vi "ReadRealStatus气密机一.vi"(0 "从站地址":u8=255 format="%x", 5 "VISA":refnum<visa-resource-name>="COM3" caption="COM", 7 "baud rate":u32=57600 caption="波特率(9600)") -> (1 "Ready":bool, 2 "Pass":bool, 3 "StepCode":u16, 4 "ProgramNumber":u16, 6 "Pressure":dbl, 8 "PressureUnit":u16(ring) items=["cm3/s"=0, "cm3/min"=1000, "cm3/h"=2000, "mm3/h"=3000, "CalibartedPascal"=4000, "Pa"=6000, "Bar"=11000, "Kpa"=12000, "PSI"=13000, "Mbar"=14000, "Mpa"=15000, "Inch3/s"=46000, "Inch3/min"=47000, "Inch3/hour"=48000], 9 "AL":bool, 10 "Leak":dbl, 11 "PressureAL":bool, 12 "RD":bool, 13 "TD":bool, 14 "StatusResults":u16 format="%b", 15 "LeakUnit":u16(ring) items=["cm3/s"=0, "cm3/min"=1000, "cm3/h"=2000, "mm3/h"=3000, "CalibartedPascal"=4000, "Pa"=6000, "Bar"=11000, "Kpa"=12000, "PSI"=13000, "Mbar"=14000, "Mpa"=15000, "Inch3/s"=46000, "Inch3/min"=47000, "Inch3/hour"=48000])   [LabVIEW 2014]
panel:
  out "Read Status":bool
  out "ReturnResultValues":u16[](array[numeric]) format="%x"
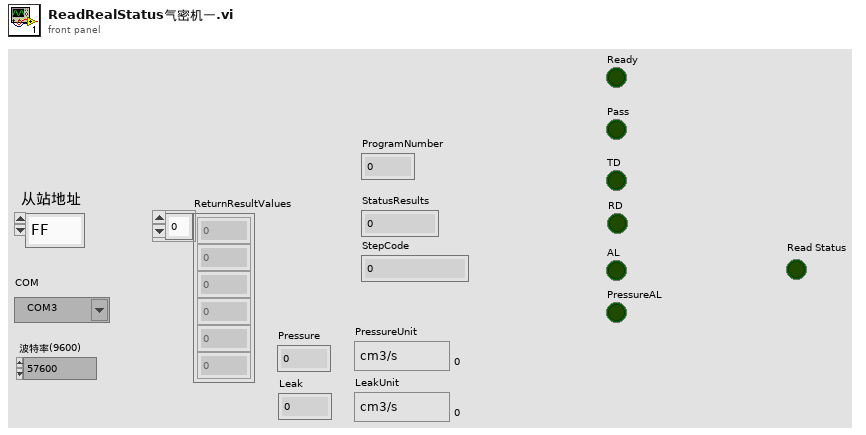
[diagram p1: front panel]
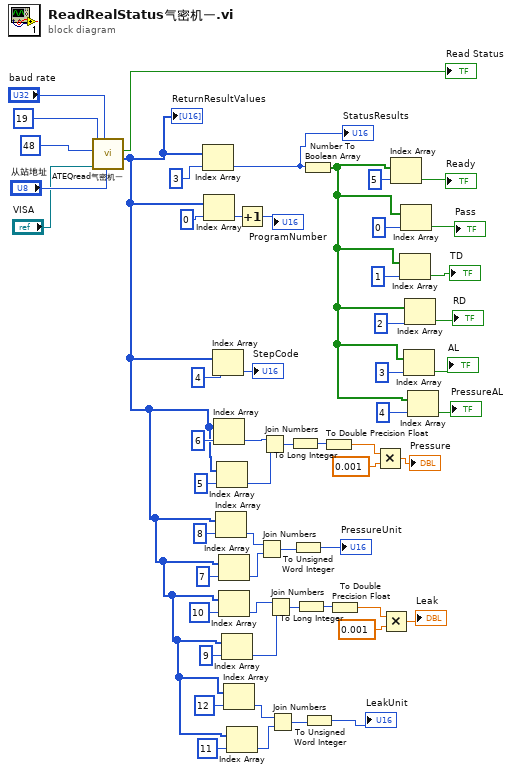
[diagram p0: block diagram]
diagram:
  n1 = call "ATEQread气密机一.vi"("baud rate (9600)"="baud rate", "VISA resource name"="VISA", "从站地址"="从站地址", "Read Address"=u16 48, "The number of Read"=u32 19) -> ("ReturnResultValues"=w12:u16[], "Read Status"=→"Read Status":bool)  [unwired: 4 in, 1 out]
  "ReturnResultValues" <- w12
  n2 = Index Array(array=w12, index=3 ("索引")) -> (element=w37:u16)
  "StatusResults" <- w37
  n3 = Index Array(array=w12, index=0 ("索引")) -> (element=w53:u16)
  n4 = Index Array(array=w12, index=4 ("索引")) -> (element=→"StepCode":u16)
  n5 = Index Array(array=w12, index=6 ("索引")) -> (element=w34:u16)
  n6 = Index Array(array=w12, index=8 ("索引")) -> (element=w26:u16)
  n7 = Index Array(array=w12, index=5 ("索引")) -> (element=w33:u16)
  n8 = Index Array(array=w12, index=7 ("索引")) -> (element=w25:u16)
  n9 = Index Array(array=w12, index=10 ("索引")) -> (element=w16:u16)
  n10 = Index Array(array=w12, index=9 ("索引")) -> (element=w15:u16)
  n11 = Index Array(array=w12, index=12 ("索引")) -> (element=w10:u16)
  n12 = Index Array(array=w12, index=11 ("索引")) -> (element=w9:u16)
  n13 = Increment(x=w53) -> (x+1=→"ProgramNumber":u16)
  n14 = Join Numbers(hi=w26, lo=w25) -> ((hi.lo)=w24:u32)
  n15 = Join Numbers(hi=w34, lo=w33) -> ((hi.lo)=w32:u32)
  n16 = Join Numbers(hi=w16, lo=w15) -> ((hi.lo)=w17:u32)
  n17 = Join Numbers(hi=w10, lo=w9) -> ((hi.lo)=w11:u32)
  n18 = To Long Integer(number=w32) -> (32bit integer=w31:i32)
  n19 = To Unsigned Word Integer(number=w24) -> (unsigned 16bit integer=→"PressureUnit":u16)
  n20 = To Long Integer(number=w17) -> (32bit integer=w18:i32)
  n21 = Number To Boolean Array(number=w37) -> (Boolean array=w3:bool[])
  n22 = To Unsigned Word Integer(number=w11) -> (unsigned 16bit integer=→"LeakUnit":u16)
  n23 = To Double Precision Float(number=w31) -> (double precision float=w29:dbl)
  n24 = To Double Precision Float(number=w18) -> (double precision float=w20:dbl)
  n25 = Multiply(x=w29, y=0.001) -> (x*y=→"Pressure":dbl)
  n26 = Multiply(x=w20, y=0.001) -> (x*y=→"Leak":dbl)
  n27 = Index Array(array=w3, index=5 ("索引")) -> (element=→"Ready":bool)
  n28 = Index Array(array=w3, index=1 ("索引")) -> (element=→"TD":bool)
  n29 = Index Array(array=w3, index=0 ("索引")) -> (element=→"Pass":bool)
  n30 = Index Array(array=w3, index=3 ("索引")) -> (element=→"AL":bool)
  n31 = Index Array(array=w3, index=2 ("索引")) -> (element=→"RD":bool)
  n32 = Index Array(array=w3, index=4 ("索引")) -> (element=→"PressureAL":bool)
